vi "Append and Sync Waveform.vi"(8 "Error":errorcluster, 9 "Waveform To Append":T1, 11 "WavBuf":refnum<class "WavBuf.lvclass">) -> (0 "Error Out":errorcluster, 3 "WavBuf Out":refnum<class "WavBuf.lvclass">)   [LabVIEW 2025, in "WavBuf.lvclass"]
uses:
  WavBuf.lvclass
  Universal Controls/Waveform_Data.ctl
  WavBuf.lvclass/WavBuf.ctl
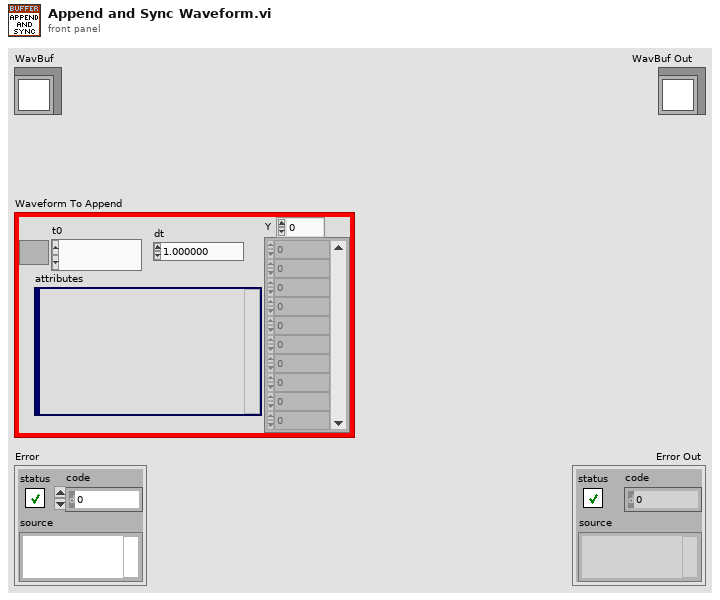
[diagram p1: front panel]
types:
  T1 = typedef "Waveform_Data.ctl" = waveform(dbl)
  T2 = typedef "Ref_DVR_Buffer.ctl" = refnum<data-value>
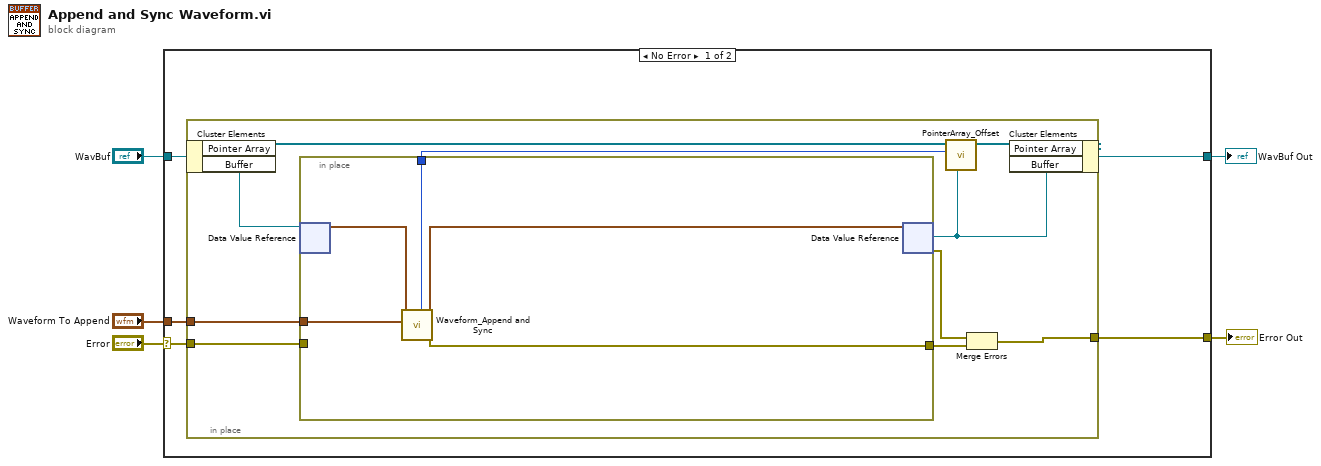
[diagram p0: block diagram]
diagram:
  n1 = case shown="No Error" "Error" {
    selector: "Error" -> [w8 w27]
    tunnel: [w6 w27] -> w4
    tunnel: [w10 w26] -> w2
    tunnel: "WavBuf" -> [w9 w26]
    tunnel: "Waveform To Append" -> [w7 _]
    frame No Error {
      n2 = in-place {
        in-place-border: w8 -> [w20]
        in-place-border: [w12] -> w6
        in-place-border: w7 -> [w19]
        n3 = in-place-cluster #1(w9) -> ("Pointer Array"=w15:refnum<class "_Pointer.lvclass">[], "Buffer"=w18:T2)
        n4 = in-place {
          in-place-border: w20 -> [_]
          in-place-border: [w22] -> w16
          in-place-border: w19 -> [w25]
          in-place-border: [w24] -> w11
          n5 = in-place-dvr #2(w18) -> (w23:T1)  [unwired: 1 out]
          n6 = call "Waveform_Append and Sync.vi"("Waveform To Append"=w25, "Waveform"=w23) -> ("Error Out"=w24:errorcluster, "Waveform Out"=w21:T1, "Offset Out"=w22:i32)  [unwired: 7 in]
          n7 = in-place-dvr #2(w21) -> (w17:T2, w13:errorcluster)
        }
        n8 = call "PointerArray_Offset.vi"("Buffer"=w17, "Total Starting Offset"=w16, "Pointer Array"=w15) -> ("Pointer Array Out"=w14:refnum<class "_Pointer.lvclass">[])  [unwired: 8 in]
        n9 = Merge Errors(w13, w11) -> (w12:errorcluster)
        n10 = in-place-cluster #1("Pointer Array"=w14, "Buffer"=w17) -> (w10:refnum<class "WavBuf.lvclass">)
      }
    }
    frame Error {
    }
  }
  "Error Out" <- w4
  "WavBuf Out" <- w2
